vi "使用者紀錄.vi"() -> ()   [LabVIEW 2015]
uses:
  <vilib>/Utility/miscctls.llb/LVRowAndColumnTypeDef.ctl
  <vilib>/Utility/miscctls.llb/LVBoundsTypeDef.ctl
  Use History.ctl
  <vilib>/Utility/miscctls.llb/LVPointTypeDef.ctl
panel:
  in  "離開":bool
  out "User Accounts Table":string[][](table)
  # "使用紀錄"
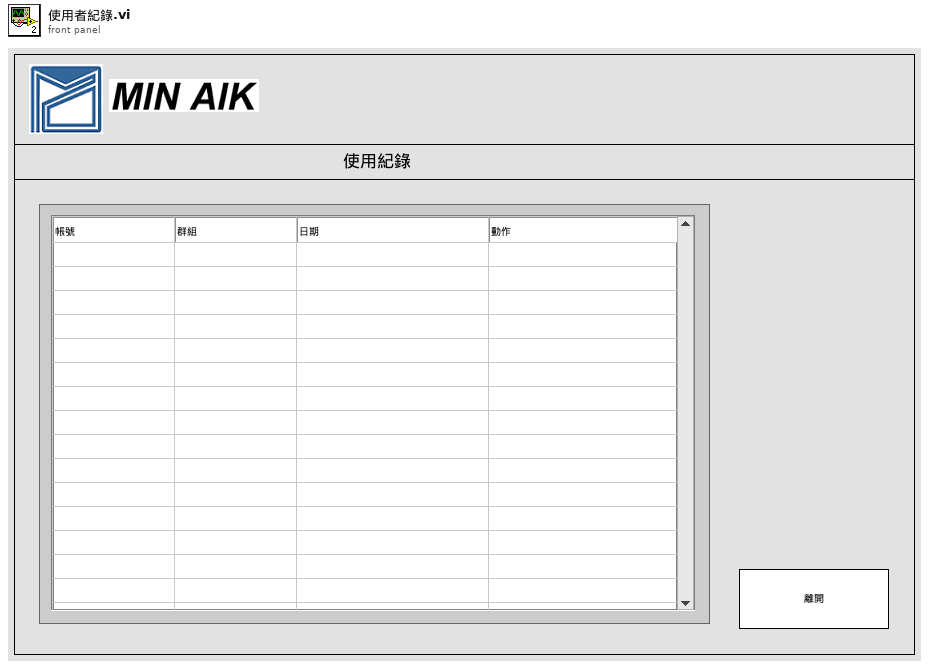
[diagram p1: front panel]
types:
  T1 = typedef "LVBoundsTypeDef.ctl" = cluster{"Width":u32, "Height":u32}
  T2 = typedef "LVRowAndColumnTypeDef.ctl" = cluster{"Row":i32, "Column":i32}
  T3 = typedef "LVPointTypeDef.ctl" = cluster{"Horizontal":i16, "Vertical":i16}
  T4 = typedef "Use History.ctl" = enum16{"Initialize", "Set Data", "Get Data", "Idle"}
  T5 = cluster{"帳號":string, "使用者等級":string, "時間":string, "事件":string}[]
  T6 = typedef "eventvkey.ctl" = enum16{"ASCII", "Enter", "Return", "Shift", "Ctrl", "Alt", "Cmd", "Opt", "Caps", "NumLock", "Clear", "Break", "Up", "Down", "Left", "Right", "Insert", "Delete", "Home", "End", "PageUp", "PageDown", "Escape", "Help", "Pause", "ScrollLock", "F1", "F2", "F3", "F4", "F5", "F6", "F7", "F8", "F9", "F10", "F11", "F12", "F13", "F14", "F15", "F16", "F17", "F18", "F19", "F20", "F21", "F22", "F23", "F24", "Play", "VolumeUp", "VolumeDown", "Mute", "Two Byte Char"}
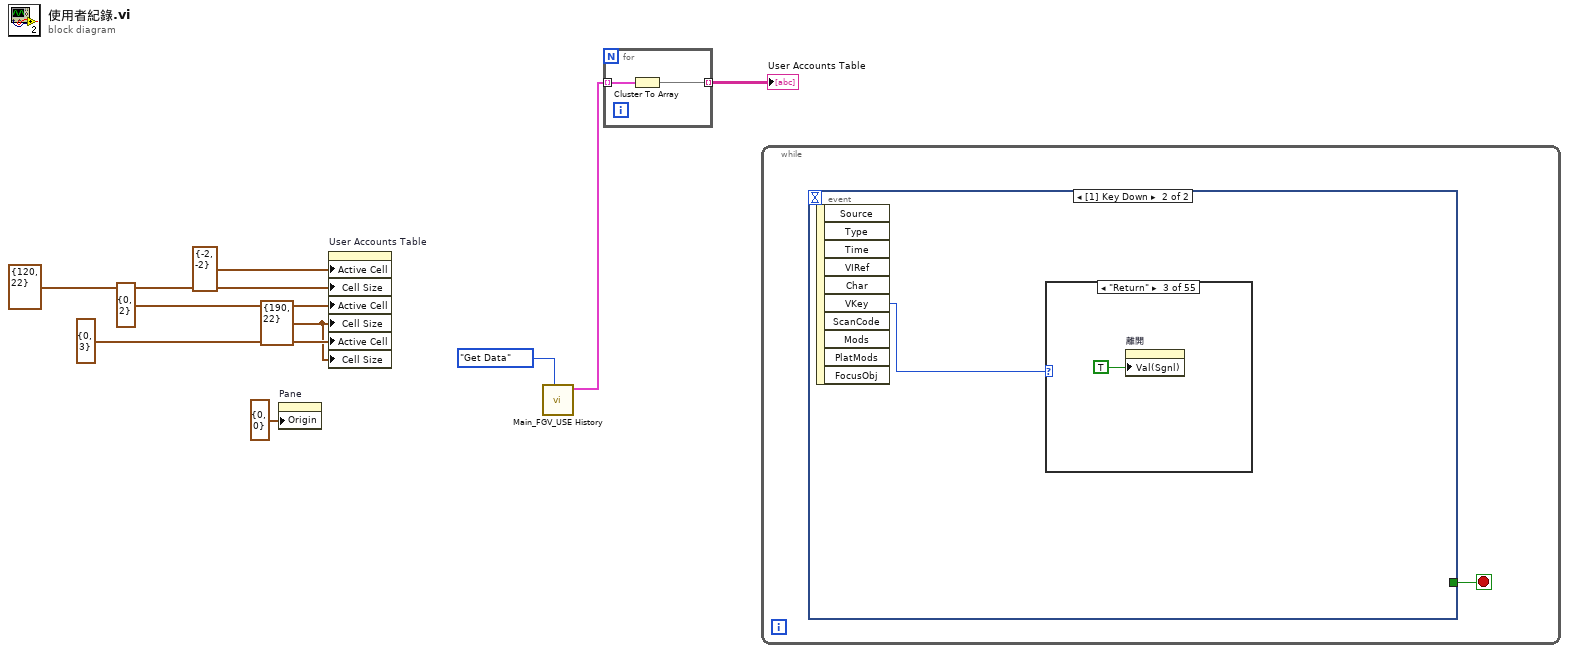
[diagram p0: block diagram]
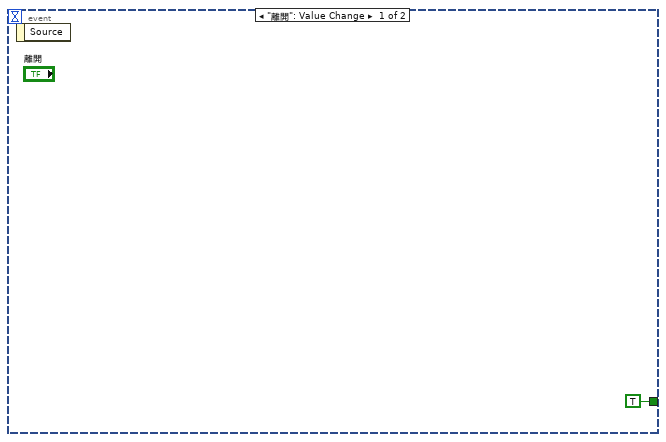
[diagram p2: hidden frame]
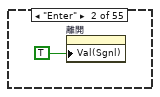
[diagram p4: hidden frame]
diagram:
  w3 = T1 {"Width"=190, "Height"=22} ("Active Cell:Cell Size")
  n1 = property on="Pane" class="Pane"("Origin"=T3 {"Horizontal"=0, "Vertical"=0}) -> ()  [unwired: 2 in, 2 out]
  n2 = property on="User Accounts Table" class="Tbl (strict)"("Active Cell"=T2 {"Row"=-2, "Column"=-2} ("Active Cell:Active Cell"), "Cell Size"=T1 {"Width"=120, "Height"=22} ("Active Cell:Cell Size"), "Active Cell"=T2 {"Row"=0, "Column"=2} ("Active Cell:Active Cell"), "Cell Size"=w3, "Active Cell"=T2 {"Row"=0, "Column"=3} ("Active Cell:Active Cell"), "Cell Size"=w3) -> ()  [unwired: 2 in, 2 out]
  n3 = call "Main_FGV_USE History.vi"("Use Action"=Use_History."Get Data") -> ("MSG Array"=w1:T5)  [unwired: 10 in]
  n4 = for {
    tunnel: w1 -> [w11] mode=indexing
    tunnel: [w10] -> w2 mode=indexing
    n5 = Cluster To Array(cluster=w11) -> (array=w10:string[])
  }
  "User Accounts Table" <- w2
  n6 = while {
    stop <- w12 stop-if-true
    n7 = event shown="[1] Key Down" {
      selector: _ -> [_ _]
      dyn-events: _ -> [_ _]
      timeout: _ -> [_ _]
      tunnel: [TRUE _] -> w12
      event "離開": Value Change {
        n8 = event-data() -> ()  [unwired: 1 in, 1 out]
      }
      event Key Down {
        n9 = event-data() -> ("VKey"=w14:T6)  [unwired: 1 in, 9 out]
        n10 = case shown="\"Return\"" w14 {
          frame "ASCII", Default {
          }
          frame "Enter" {
            n11 = property on="離開" class="Bool (strict)"("Val(Sgnl)"=TRUE ("Value (Signaling)")) -> ()  [unwired: 2 in, 2 out]
          }
          frame "Return" {
            n12 = property on="離開" class="Bool (strict)"("Val(Sgnl)"=TRUE ("Value (Signaling)")) -> ()  [unwired: 2 in, 2 out]
          }
          frame "Shift" {
          }
          frame "Ctrl" {
          }
          frame "Alt" {
          }
          frame "Cmd" {
          }
          frame "Opt" {
          }
          frame "Caps" {
          }
          frame "NumLock" {
          }
          frame "Clear" {
          }
          frame "Break" {
          }
          frame "Up" {
          }
          frame "Down" {
          }
          frame "Left" {
          }
          frame "Right" {
          }
          frame "Insert" {
          }
          frame "Delete" {
          }
          frame "Home" {
          }
          frame "End" {
          }
          frame "PageUp" {
          }
          frame "PageDown" {
          }
          frame "Escape" {
          }
          frame "Help" {
          }
          frame "Pause" {
          }
          frame "ScrollLock" {
          }
          frame "F1" {
          }
          frame "F2" {
          }
          frame "F3" {
          }
          frame "F4" {
          }
          frame "F5" {
          }
          frame "F6" {
          }
          frame "F7" {
          }
          frame "F8" {
          }
          frame "F9" {
          }
          frame "F10" {
          }
          frame "F11" {
          }
          frame "F12" {
          }
          frame "F13" {
          }
          frame "F14" {
          }
          frame "F15" {
          }
          frame "F16" {
          }
          frame "F17" {
          }
          frame "F18" {
          }
          frame "F19" {
          }
          frame "F20" {
          }
          frame "F21" {
          }
          frame "F22" {
          }
          frame "F23" {
          }
          frame "F24" {
          }
          frame "Play" {
          }
          frame "VolumeUp" {
          }
          frame "VolumeDown" {
          }
          frame "Mute" {
          }
          frame "Two Byte Char" {
          }
        }
      }
    }
  }
